vi "testGetInstanceGenServersAandB.vi"(8 "error in (no error)":errorcluster) -> (0 "error out":errorcluster)   [LabVIEW 2018]
uses:
  src/TcpServer/TcpServer.lvclass
  <vilib>/addons/_JKI Toolkits/Caraya/classes/Assert/Assert Not Equal Value_Variant.vi
  <vilib>/addons/_JKI Toolkits/Caraya/classes/Test/Test.lvclass
  <vilib>/addons/_JKI Toolkits/Caraya/classes/Assert/Assert.lvclass
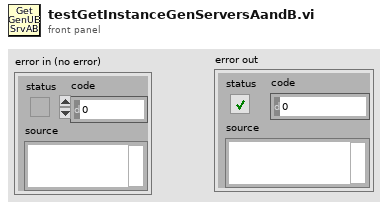
[diagram p1: front panel]
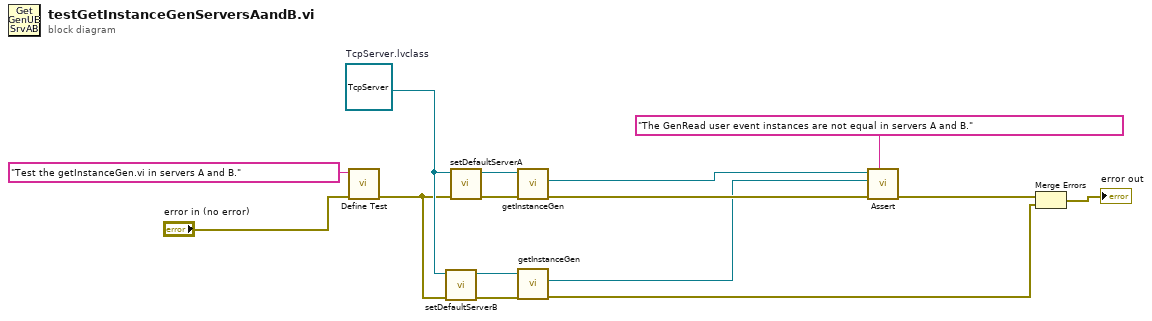
[diagram p0: block diagram]
diagram:
  w9 = refnum<class "TcpServer.lvclass"> refnum  # TcpServer.lvclass
  n1 = call <vilib>:"Define Test.vi"("error in (no error)"="error in (no error)", "Label (VI Title)"="Test the getInstanceGen.vi in servers A and B.") -> ("error out"=w8:errorcluster)  [unwired: 9 in]
  n2 = call "setDefaultServerB.vi"("error in (no error)"=w8, "TcpServer.lvclass"=w9) -> ("error out"=w6:errorcluster, "tcpServer out"=w7:refnum<class "TcpServer.lvclass">)  [unwired: 8 in]
  n3 = call "setDefaultServerA.vi"("error in (no error)"=w8, "TcpServer.lvclass"=w9) -> ("error out"=w12:errorcluster, "tcpServer out"=w13:refnum<class "TcpServer.lvclass">)  [unwired: 8 in]
  n4 = call "getInstanceGen.vi"("error in (no error)"=w12, "tcpServer in"=w13) -> ("error out"=w10:errorcluster, "GenRead"=w4:refnum<user-event>)  [unwired: 7 in, 1 out]
  n5 = call "getInstanceGen.vi"("error in (no error)"=w6, "tcpServer in"=w7) -> ("error out"=w2:errorcluster, "GenRead"=w3:refnum<user-event>)  [unwired: 7 in, 1 out]
  n6 = call-poly <vilib>:"Assert.vi"("Label"="The GenRead user event instances are not equal in servers A and B." ("Label (VI Title)"), "error in (no error)"=w10, "Y"=w3, "X"=w4) -> ("error out"=w11:errorcluster)  [unwired: 7 in]
  n7 = Merge Errors(w11, w2) -> (→"error out":errorcluster)
